vi "read station nvh config.vi"(8 "error in":errorcluster, 10 "station idx":i32, 11 "configuration file path in":path) -> (0 "error out":errorcluster, 2 "st nvh config":T1, 3 "configuration file path out":path)   [LabVIEW 2018]
uses:
  02.Type Def's/station nvh config.ctl
  05.UserVI's/file io/ini/type defs/ini file actions.ctl
  05.UserVI's/file io/ini/type defs/ini entry value.ctl
  05.UserVI's/file io/ini/type defs/ini entry types.ctl
  05.UserVI's/file io/ini/type defs/ini entry.ctl
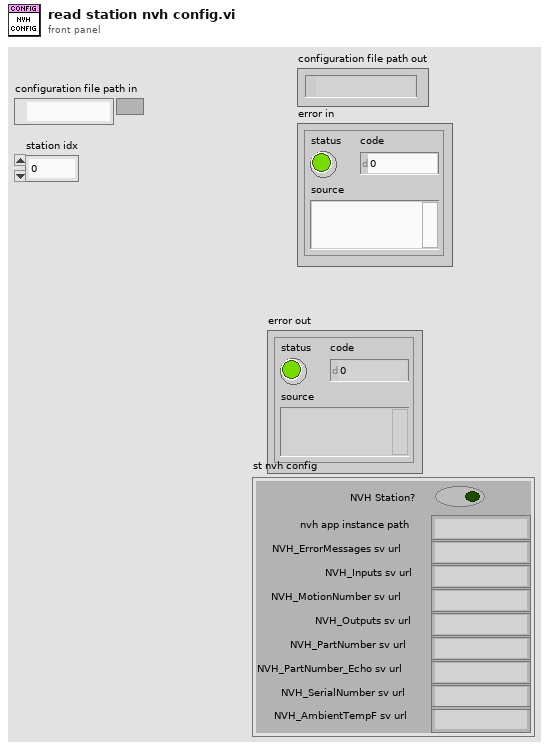
[diagram p1: front panel]
types:
  T1 = typedef "station nvh config.ctl" = cluster{"NVH Station?":bool, "nvh app instance path":string, "NVH_ErrorMessages sv url":string, "NVH_Inputs sv url":string, "NVH_MotionNumber sv url":string, "NVH_Outputs sv url":string, "NVH_PartNumber sv url":string, "NVH_PartNumber_Echo sv url":string, "NVH_SerialNumber sv url":string, "NVH_AmbientTempF sv url":string}
  T2 = typedef "ini entry value.ctl" = cluster{"Boolean":bool, "Dbl":dbl, "I32":i32, "Path":path, "String":string, "U32":u32}
  T3 = typedef "ini file actions.ctl" = enum16{"read ini", "write ini"}
  T4 = typedef "ini entry.ctl" = cluster{"section":string, "key":string, "type":T5, "default value":T2}
  T5 = typedef "ini entry types.ctl" = enum16{"Boolean", "Double", "I32", "Path", "String", "U32"}
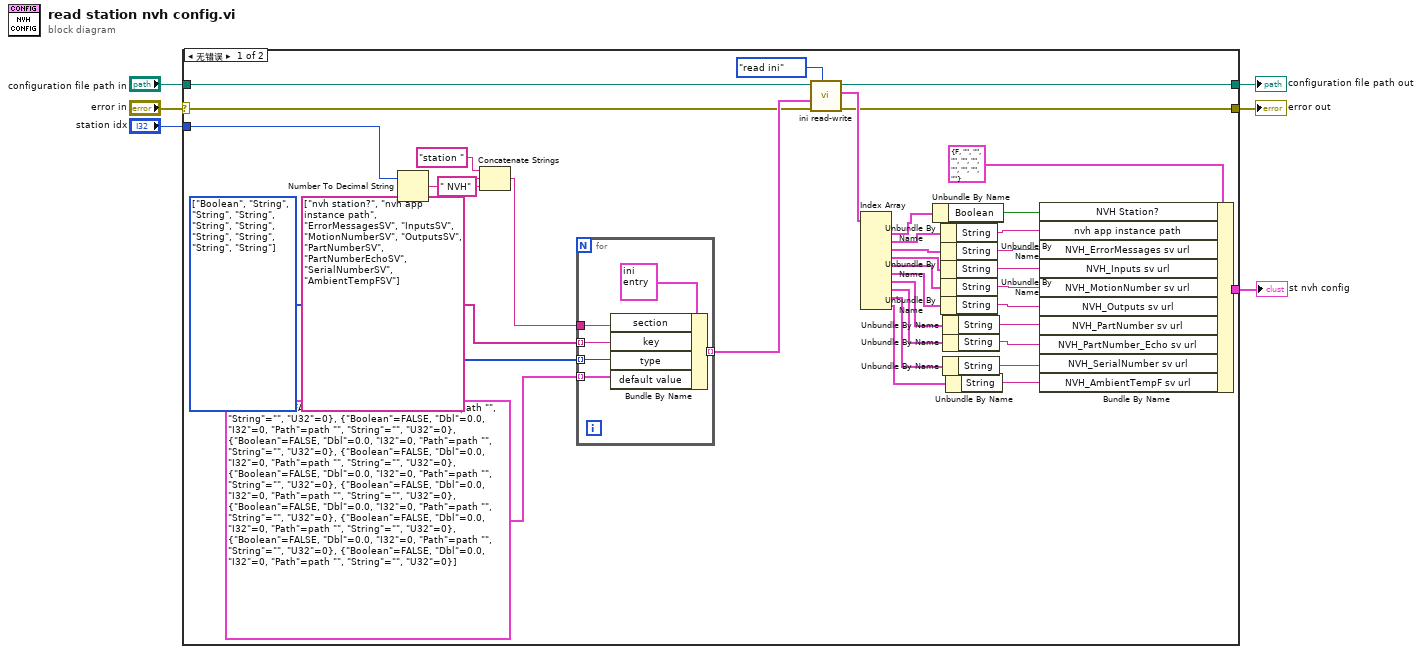
[diagram p0: block diagram]
diagram:
  n1 = case shown="无错误" "error in" {
    selector: "error in" -> [w25 w51]
    tunnel: "configuration file path in" -> [w43 w50]
    tunnel: [w38 w50] -> w5
    tunnel: [w37 w51] -> w4
    tunnel: "station idx" -> [w35 _]
    tunnel: [w22 _] -> w1
    frame No Error {
      w28 = T5[] [enum."Boolean", enum."String", enum."String", enum."String", enum."String", enum."String", enum."String", enum."String", enum."String", enum."String"] items=["Boolean", "Double", "I32", "Path", "String", "U32"]
      n2 = Number To Decimal String(number=w35) -> (decimal integer string=w34:string)  [unwired: 1 in]
      n3 = Concatenate Strings("station ", w34, " NVH" ("string")) -> (w33:string)
      n4 = for {
        tunnel: w33 -> [w48]
        tunnel: string[] ["nvh station?", "nvh app instance path", "ErrorMessagesSV", "InputsSV", "MotionNumberSV", "OutputsSV", "PartNumberSV", "PartNumberEchoSV", "SerialNumberSV", "AmbientTempFSV"] -> [w47] mode=indexing
        tunnel: w28 -> [w46] mode=indexing
        tunnel: T2[] [{"Boolean"=FALSE, "Dbl"=0.0, "I32"=0, "Path"=path "", "String"="", "U32"=0}, {"Boolean"=FALSE, "Dbl"=0.0, "I32"=0, "Path"=path "", "String"="", "U32"=0}, {"Boolean"=FALSE, "Dbl"=0.0, "I32"=0, "Path"=path "", "String"="", "U32"=0}, {"Boolean"=FALSE, "Dbl"=0.0, "I32"=0, "Path"=path "", "String"="", "U32"=0}, {"Boolean"=FALSE, "Dbl"=0.0, "I32"=0, "Path"=path "", "String"="", "U32"=0}, {"Boolean"=FALSE, "Dbl"=0.0, "I32"=0, "Path"=path "", "String"="", "U32"=0}, {"Boolean"=FALSE, "Dbl"=0.0, "I32"=0, "Path"=path "", "String"="", "U32"=0}, {"Boolean"=FALSE, "Dbl"=0.0, "I32"=0, "Path"=path "", "String"="", "U32"=0}, {"Boolean"=FALSE, "Dbl"=0.0, "I32"=0, "Path"=path "", "String"="", "U32"=0}, {"Boolean"=FALSE, "Dbl"=0.0, "I32"=0, "Path"=path "", "String"="", "U32"=0}] -> [w45] mode=indexing
        tunnel: [w44] -> w26 mode=indexing
        n5 = Bundle By Name(cluster=T4 {"section"="", "key"="", "type"=enum."Boolean", "default value"={"Boolean"=FALSE, "Dbl"=0.0, "I32"=0, "Path"=path "", "String"="", "U32"=0}}, "section"=w48, "key"=w47, "type"=w46, "default value"=w45) -> (w44:T4)
      }
      n6 = call "ini read-write.vi"("action"=ini_file_actions."read ini", "error in (no error)"=w25, "ini entry descriptors"=w26, "configuration file path"=w43) -> ("error out"=w37:errorcluster, "values out"=w41:T2[], "configuration file path out"=w38:path)  [unwired: 5 in]
      n7 = Index Array(array=w41) -> (element #1=w21:T2, element #2=w40:T2, element #3=w39:T2, element #4=w32:T2, element #5=w31:T2, element #6=w30:T2, element #7=w11:T2, element #8=w10:T2, element #9=w9:T2, element #10=w8:T2)  [unwired: 10 in]
      n8 = Unbundle By Name(w21) -> ("Boolean"=w20:bool)
      n9 = Unbundle By Name(w40) -> ("String"=w19:string)
      n10 = Unbundle By Name(w39) -> ("String"=w18:string)
      n11 = Unbundle By Name(w32) -> ("String"=w17:string)
      n12 = Unbundle By Name(w31) -> ("String"=w16:string)
      n13 = Unbundle By Name(w30) -> ("String"=w15:string)
      n14 = Unbundle By Name(w11) -> ("String"=w14:string)
      n15 = Unbundle By Name(w10) -> ("String"=w13:string)
      n16 = Unbundle By Name(w9) -> ("String"=w12:string)
      n17 = Unbundle By Name(w8) -> ("String"=w7:string)
      n18 = Bundle By Name(cluster=T1 {"NVH Station?"=FALSE, "nvh app instance path"="", "NVH_ErrorMessages sv url"="", "NVH_Inputs sv url"="", "NVH_MotionNumber sv url"="", "NVH_Outputs sv url"="", "NVH_PartNumber sv url"="", "NVH_PartNumber_Echo sv url"="", "NVH_SerialNumber sv url"="", "NVH_AmbientTempF sv url"=""} ("NVH Configuration"), "NVH Station?"=w20, "nvh app instance path"=w19, "NVH_ErrorMessages sv url"=w18, "NVH_Inputs sv url"=w17, "NVH_MotionNumber sv url"=w16, "NVH_Outputs sv url"=w15, "NVH_PartNumber sv url"=w14, "NVH_PartNumber_Echo sv url"=w13, "NVH_SerialNumber sv url"=w12, "NVH_AmbientTempF sv url"=w7) -> (w22:T1)
    }
    frame Error {
    }
  }
  "configuration file path out" <- w5
  "error out" <- w4
  "st nvh config" <- w1
